vi "Init OLED.vi"(8 "error in (no error)":errorcluster, 11 "48x64 I2C OLED SSD1306 in":refnum<class "48x64 I2C OLED SSD1306.lvclass">) -> (0 "error out":errorcluster, 2 "2D Picture":picture, 3 "48x64 I2C OLED SSD1306 out":refnum<class "48x64 I2C OLED SSD1306.lvclass">)   [LabVIEW 2020, in "CTI-Peripheral.lvlib" / "48x64 I2C OLED SSD1306.lvclass"]
uses:
  48x64 I2C OLED SSD1306.lvclass
  48x64 I2C OLED SSD1306.lvclass/48x64 I2C OLED SSD1306.ctl
  CTI/I2C Connection/I2C Connection.lvclass/I2C Connection.ctl
  InitialiseOLED.vi
  CTI/Session/I2C Write Data.vi
  CTI/I2C Connection/I2C Connection.lvclass
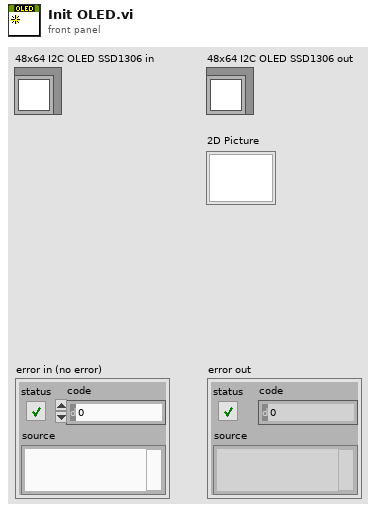
[diagram p1: front panel]
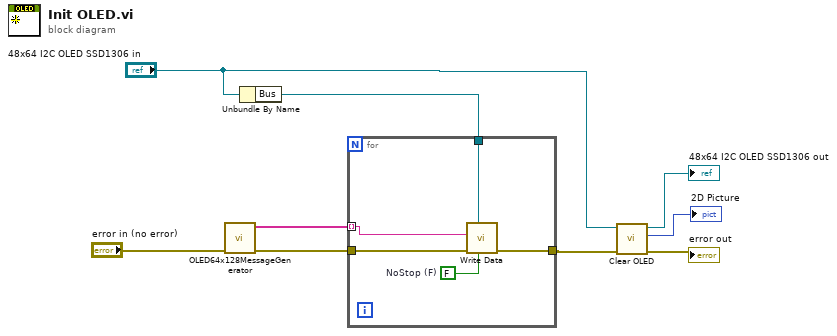
[diagram p0: block diagram]
diagram:
  n1 = call-poly "OLED64x128MessageGenerator.vi"("error in (no error)"="error in (no error)") -> ("error out"=w8:errorcluster, "Messages"=w6:string[])  [unwired: 9 in]
  n2 = Unbundle By Name("48x64 I2C OLED SSD1306 in") -> ("Bus"=w9:refnum<class "I2C Connection.lvclass">)
  n3 = for {
    tunnel: w9 -> [w13]
    tunnel: w6 -> [w10] mode=indexing
    tunnel: w8 -> [w11]
    tunnel: [w14] -> w5
    w12 = FALSE  # NoStop (F)
    n4 = call "Write Data.vi"("NoStop (F)"=w12, "I2C Connection"=w13, "error in (no error)"=w11, "Data"=w10) -> ("error out"=w14:errorcluster)  [unwired: 7 in]
  }
  n5 = call "Clear OLED.vi"("error in (no error)"=w5, "64x128 I2C OLED SSD1315 in"="48x64 I2C OLED SSD1306 in") -> ("error out"=→"error out":errorcluster, "2D Picture"=→"2D Picture":picture, "64x128 I2C OLED SSD1315 out"=→"48x64 I2C OLED SSD1306 out":refnum<class "48x64 I2C OLED SSD1306.lvclass">)  [unwired: 7 in]
